vi "Set.vi"(10 "Value":refnum<class "Entity.lvclass">, 11 "Entity in":refnum<class "Entity.lvclass">) -> (3 "Entity out":refnum<class "Entity.lvclass">)   [LabVIEW 2020, in "Conditu2.lvlib" / "Columns.lvlib" / "Entity.lvclass"]
uses:
  Entity.lvclass
  Entity/Entity.lvclass
  Entity.lvclass/Entity.ctl
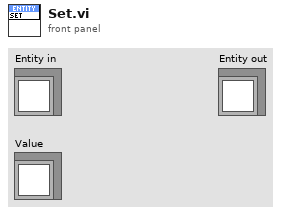
[diagram p1: front panel]
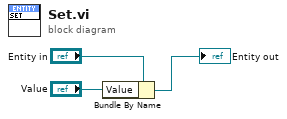
[diagram p0: block diagram]
diagram:
  n1 = Bundle By Name(cluster="Entity in", "Value"="Value") -> (→"Entity out":refnum<class "Entity.lvclass">)
